vi "InstrumentSelection.vi"(8 "error in (no error)":errorcluster, 10 "Instrument type":u16(ring) items=["Supply", "LCR"], 11 "Instrument name IN":string(combo)) -> (0 "error out":errorcluster, 1 "Instrument name OUT":string, 2 "LCR":refnum<class "LCRControl.lvclass">, 3 "Supply":refnum<class "SupplyControl.lvclass">)   [LabVIEW 2013]
uses:
  SupplyControl/SupplyControl.lvclass
  LCRControl/LCRControl.lvclass
  SupplyControl/Keithley 2410/KE2410.lvclass
  SupplyControl/Keithley 6517/KE6517.lvclass
  SupplyControl/Keithley 487/KE487.lvclass
  LCRControl/WK6440B/WK6440B.lvclass
  InstrControl.lvclass
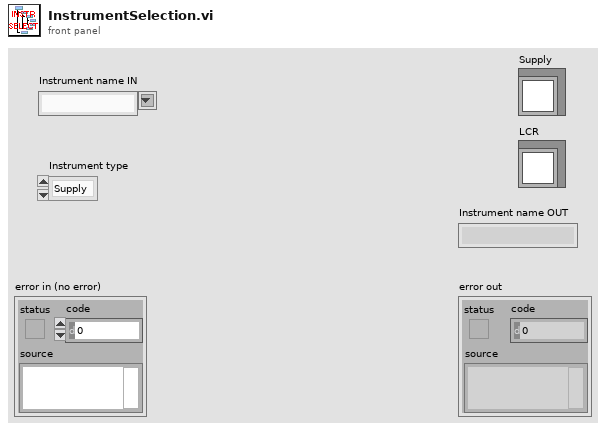
[diagram p1: front panel]
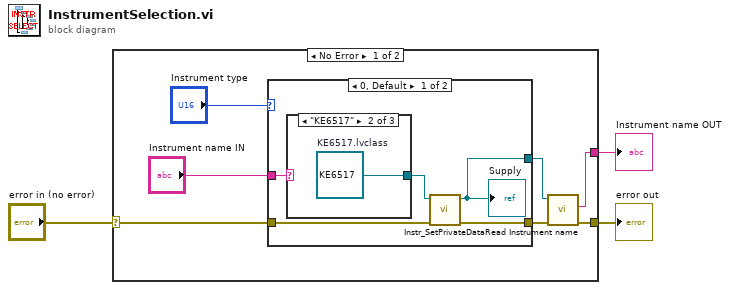
[diagram p0: block diagram]
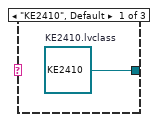
[diagram p2: hidden frame]
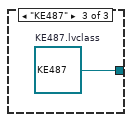
[diagram p3: hidden frame]
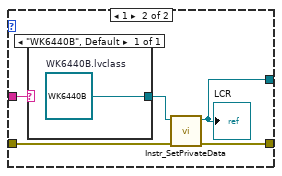
[diagram p4: hidden frame]
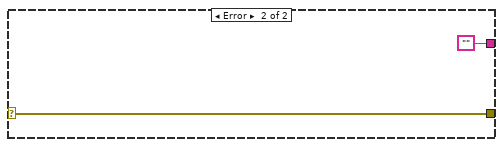
[diagram p5: hidden frame]
diagram:
  n1 = case shown="No Error" "error in (no error)" {
    selector: "error in (no error)" -> [w6 w26]
    tunnel: [w7 w26] -> w2
    tunnel: [w8 ""] -> w1
    frame No Error {
      n2 = case shown="0, Default" "Instrument type" {
        tunnel: "Instrument name IN" -> [w15 w23]
        tunnel: [w13 w21] -> w5
        tunnel: w6 -> [w11 w20]
        tunnel: [w12 w19] -> w4
        frame 0, Default {
          n3 = case shown="\"KE6517\"" w15 {
            tunnel: [w16 w17 w18] -> w14
            frame "KE2410", Default {
              w16 = refnum<class "KE2410.lvclass"> refnum  # KE2410.lvclass
            }
            frame "KE6517" {
              w17 = refnum<class "KE6517.lvclass"> refnum  # KE6517.lvclass
            }
            frame "KE487" {
              w18 = refnum<class "KE487.lvclass"> refnum  # KE487.lvclass
            }
          }
          n4 = call-dynamic "Instr_SetPrivateData.vi"("error in (no error)"=w11, "SupplyControl in"=w14) -> ("error out"=w12:errorcluster, "SupplyControl out"=w13:refnum<class "SupplyControl.lvclass">)  [unwired: 8 in]
          "Supply" <- w13
        }
        frame 1 {
          n5 = case shown="\"WK6440B\", Default" w23 {
            tunnel: [w24] -> w22
            frame "WK6440B", Default {
              w24 = refnum<class "WK6440B.lvclass"> refnum  # WK6440B.lvclass
            }
          }
          n6 = call-dynamic "Instr_SetPrivateData.vi"("error in (no error)"=w20, "WK6440B in"=w22) -> ("error out"=w19:errorcluster, "WK6440B out"=w21:refnum<class "WK6440B.lvclass">)  [unwired: 8 in]
          "LCR" <- w21
        }
      }
      n7 = call-dynamic "Read Instrument name.vi"("error in (no error)"=w4, "InstControl in"=w5) -> ("error out"=w7:errorcluster, "Instrument name"=w8:string)  [unwired: 7 in, 1 out]
    }
    frame Error {
    }
  }
  "error out" <- w2
  "Instrument name OUT" <- w1
